vi "Paired t-test.vi"(6 "POST":dbl[](array[numeric])=[4930.0, 4900.0, 5140.0, 5700.0, 6110.0, 6880.0, 7930.0, 5010.0], 7 "PRE":dbl[](array[numeric])=[4900.0, 5220.0, 5500.0, 6020.0, 6340.0, 7660.0, 8650.0, 4870.0]) -> (3 "t-Test Statistics":cluster{"t-Value":dbl, "DF":i32, "P-value":dbl})   [LabVIEW 2017]
uses:
  <vilib>/gmath/statdist.llb/Student t CDF.vi
  <vilib>/Analysis/NI_AALBase.lvlib
  <vilib>/gmath/NI_Gmath.lvlib
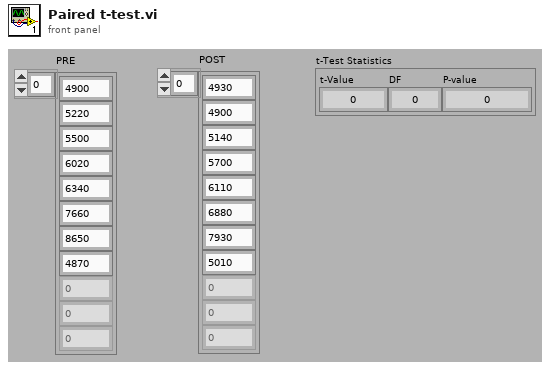
[diagram p1: front panel]
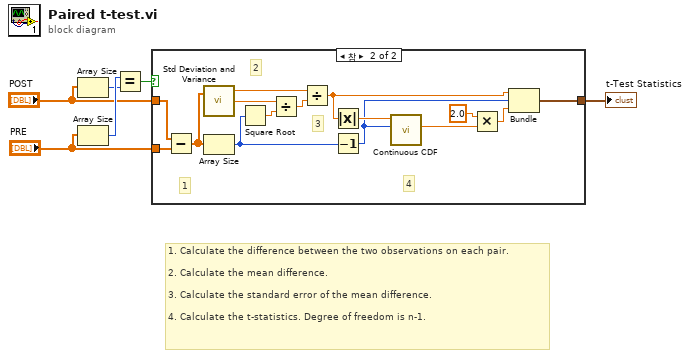
[diagram p0: block diagram]
diagram:
  # "1. Calculate the difference between the two observations on each pair.\n\n2. Calculate the mean difference.\n\n3. Calculate the standard error of the mean difference. \n\n4. Calculate the t-statistics. Degree of freedom is n-1."
  n1 = Array Size(array="POST") -> (size(s)=w5:i32)
  n2 = Array Size(array="PRE") -> (size(s)=w6:i32)
  n3 = Equal?(x=w6, y=w5) -> (x = y?=w4:bool)
  n4 = case shown="참" w4 {
    tunnel: "PRE" -> [_ w9]
    tunnel: "POST" -> [_ w10]
    tunnel: [_ w7] -> w1
    frame False {
    }
    frame True {
      # "4"
      # "3"
      # "2"
      # "1"
      n5 = Subtract(x=w10, y=w9) -> (x-y=w8:dbl[])
      n6 = call <vilib>:"Std Deviation and Variance.vi"("X"=w8) -> ("mean"=w19:dbl, "standard deviation"=w21:dbl)  [unwired: 1 in, 1 out]
      n7 = Array Size(array=w8) -> (size(s)=w17:i32)
      n8 = Square Root(x=w17) -> (sqrt(x)=w20:dbl)
      n9 = Divide(x=w21, y=w20) -> (x/y=w18:dbl)
      n10 = Divide(x=w19, y=w18) -> (x/y=w13:dbl)
      n11 = Absolute Value(x=w13) -> (abs(x)=w16:dbl)
      n12 = Decrement(x=w17) -> (x-1=w12:i32)
      n13 = call-poly <vilib>:"Continuous CDF.vi"("k degrees of freedom"=w12, "x"=w16) -> ("1-cdf(x)"=w15:dbl)  [unwired: 7 in, 2 out]
      n14 = Multiply(x=2.0, y=w15) -> (x*y=w11:dbl)
      n15 = Bundle(w13, w12, w11) -> (w7:cluster{dbl, i32, dbl})  [unwired: 1 in]
    }
  }
  "t-Test Statistics" <- w1
